vi "Check LM Buffer.vi"(8 "error in (no error)":errorcluster, 10 "SLAM In":T1, 11 "Observed LM Array":T3(array[cluster])) -> (0 "error out":errorcluster, 2 "SLAM Out":T1)   [LabVIEW 2009]
uses:
  Controls/SLAM.ctl
  <vilib>/Analysis/Matrix/Datatypes/RealMatrix.ctl
  cRIO/Functional Global Variables/Actions for FG's.ctl
  <vilib>/Analysis/Matrix/NI_Matrix.lvlib
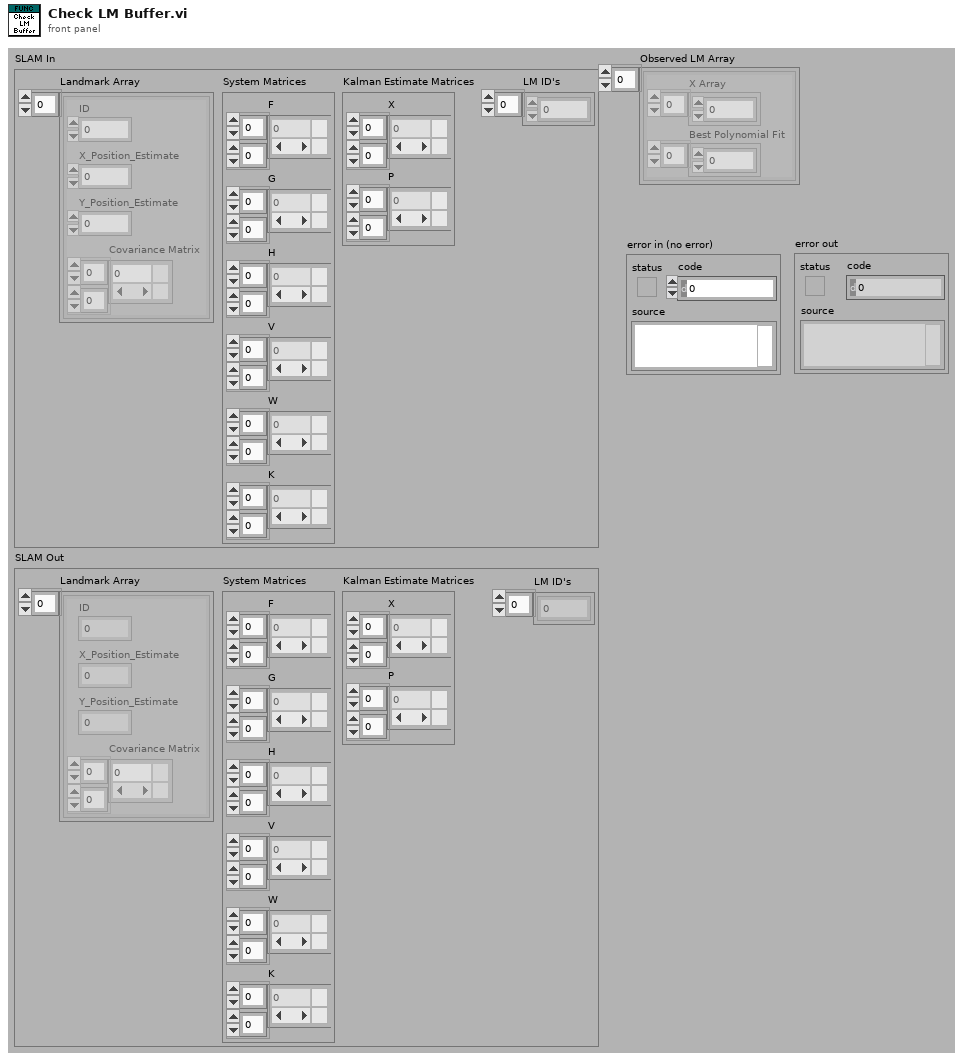
[diagram p1: front panel]
types:
  T1 = typedef "SLAM.ctl" = cluster{"Landmark Array":cluster{"ID":dbl, "X_Position_Estimate":dbl, "Y_Position_Estimate":dbl, "Covariance Matrix":T2}[], "System Matrices":cluster{"F":T2, "G":T2, "H":T2, "V":T2, "W":T2, "K":T2}, "Kalman Estimate Matrices":cluster{"X":T2, "P":T2}, "LM ID's":dbl[]}
  T2 = typedef "NI_Matrix.lvlib/RealMatrix.ctl" = dbl[][]
  T3 = cluster{"X Array":dbl[], "Best Polynomial Fit":dbl[]}[]
  T4 = typedef "Actions for FG's.ctl" = enum16{"Read", "Write"}
  T5 = cluster{"ID":dbl, "X_Position_Estimate":dbl, "Y_Position_Estimate":dbl, "Covariance Matrix":T2}[]
  T6 = cluster{"ID":dbl, "X_Position_Estimate":dbl, "Y_Position_Estimate":dbl, "Covariance Matrix":T2}
  T7 = cluster{"X Array":dbl[], "Best Polynomial Fit":dbl[], "Times Observed":dbl, "Times Not Observed":dbl}[]
  T8 = cluster{"X Array":dbl[], "Best Polynomial Fit":dbl[], "Times Observed":dbl, "Times Not Observed":dbl}
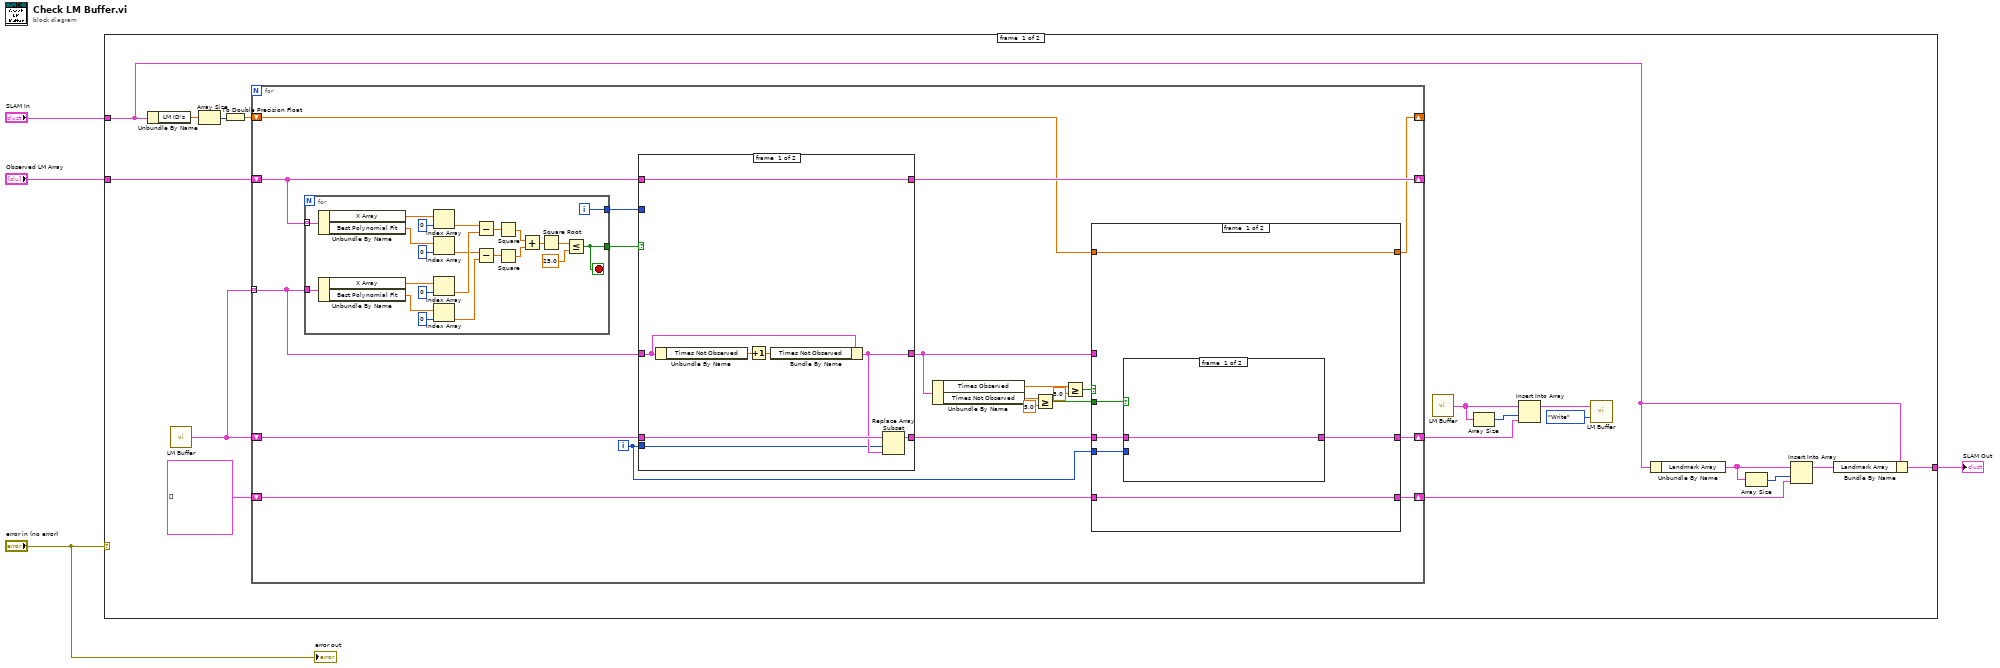
[diagram p0: block diagram]
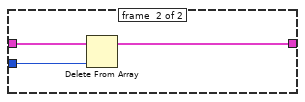
[diagram p2: hidden frame]
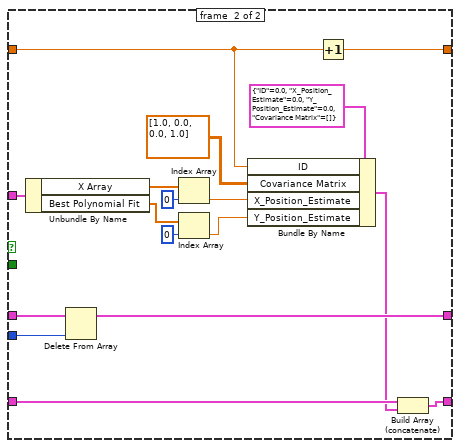
[diagram p3: hidden frame]
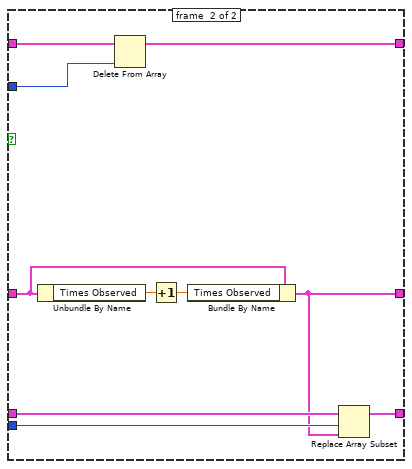
[diagram p4: hidden frame]
diagram:
  n1 = case shown="No Error" "error in (no error)" {
    tunnel: "Observed LM Array" -> [w19 _]
    tunnel: "SLAM In" -> [w7 _]
    tunnel: [w5 _] -> w2
    frame #0 {
      n2 = Unbundle By Name(w7) -> ("LM ID's"=w18:dbl[])
      n3 = call "LM Buffer.vi"() -> ("LM Buffer Out"=w21:T7)  [unwired: 2 in]
      n4 = Array Size(array=w18) -> (size(s)=w17:i32)
      n5 = To Double Precision Float(number=w17) -> (double precision float=w16:dbl)
      n6 = for {
        shift-right: [w38] -> _
        shift-left: w19 -> [w40]
        shift-right: [w30] -> w13
        shift-left: w21 -> [w27]
        shift-right: [w22] -> w8
        shift-left: T5 [] ("Landmark Array") -> [w29]
        tunnel: w21 -> [w28] mode=indexing
        shift-right: [w23] -> _
        shift-left: w16 -> [w24]
        i -> [w25]
        n7 = for {
          tunnel: w28 -> [w109]
          tunnel: w40 -> [w93] mode=indexing
          tunnel: [w95] -> w41
          tunnel: [w94] -> w39
          i -> [w94]
          stop <- w95 stop-if-true
          n8 = Unbundle By Name(w93) -> ("X Array"=w90:dbl[], "Best Polynomial Fit"=w89:dbl[])
          n9 = Unbundle By Name(w109) -> ("X Array"=w106:dbl[], "Best Polynomial Fit"=w105:dbl[])
          n10 = Index Array(array=w90, index=0) -> (element=w88:dbl)
          n11 = Index Array(array=w89, index=0) -> (element=w87:dbl)
          n12 = Index Array(array=w106, index=0) -> (element=w97:dbl)
          n13 = Index Array(array=w105, index=0) -> (element=w96:dbl)
          n14 = Subtract(x=w88, y=w97) -> (x-y=w99:dbl)
          n15 = Subtract(x=w87, y=w96) -> (x-y=w98:dbl)
          n16 = Square(x=w99) -> (x^2=w100:dbl)
          n17 = Square(x=w98) -> (x^2=w101:dbl)
          n18 = Add(x=w100, y=w101) -> (x+y=w102:dbl)
          n19 = Square Root(x=w102) -> (sqrt(x)=w103:dbl)
          n20 = Less Or Equal?(x=w103, y=25.0) -> (x <= y?=w95:bool)
        }
        n21 = case shown="True" w41 {
          tunnel: w28 -> [w73 w86]
          tunnel: [w70 w77] -> w32
          tunnel: w40 -> [w76 w83]
          tunnel: w39 -> [_ w82]
          tunnel: [w76 w81] -> w38
          tunnel: w27 -> [w72 w80]
          tunnel: w25 -> [w69 w79]
          tunnel: [w71 w78] -> w26
          frame #0 {
            n22 = Unbundle By Name(w73) -> ("Times Not Observed"=w74:dbl)
            n23 = Increment(x=w74) -> (x+1=w75:dbl)
            n24 = Bundle By Name(cluster=w73, "Times Not Observed"=w75) -> (w70:T8)
            n25 = Replace Array Subset(array=w72, new element=w70, index=w69) -> (w71:T7)
          }
          frame #1 {
            n26 = Unbundle By Name(w86) -> ("Times Observed"=w84:dbl)
            n27 = Delete From Array(array=w83, index=w82) -> (array with subset deleted=w81:T3)  [unwired: 1 in, 1 out]
            n28 = Increment(x=w84) -> (x+1=w85:dbl)
            n29 = Bundle By Name(cluster=w86, "Times Observed"=w85) -> (w77:T8)
            n30 = Replace Array Subset(array=w80, new element=w77, index=w79) -> (w78:T7)
          }
        }
        n31 = Unbundle By Name(w32) -> ("Times Observed"=w37:dbl, "Times Not Observed"=w34:dbl)
        n32 = Greater Or Equal?(x=w34, y=5.0) -> (x >= y?=w31:bool)
        n33 = Greater Or Equal?(x=w37, y=5.0) -> (x >= y?=w33:bool)
        n34 = case shown="True" w33 {
          tunnel: w32 -> [_ w68]
          tunnel: w31 -> [w47 _]
          tunnel: w26 -> [w45 w67]
          tunnel: w25 -> [w46 w66]
          tunnel: [w44 w65] -> w30
          tunnel: w29 -> [w42 w64]
          tunnel: w24 -> [w43 w55]
          tunnel: [w43 w54] -> w23
          tunnel: [w42 w52] -> w22
          frame #0 {
            n35 = case shown="True" w47 {
              tunnel: w46 -> [_ w51]
              tunnel: w45 -> [w48 w50]
              tunnel: [w48 w49] -> w44
              frame #0 {
              }
              frame #1 {
                n36 = Delete From Array(array=w50, index=w51) -> (array with subset deleted=w49:T7)  [unwired: 1 in, 1 out]
              }
            }
          }
          frame #1 {
            n37 = Unbundle By Name(w68) -> ("X Array"=w61:dbl[], "Best Polynomial Fit"=w60:dbl[])
            n38 = Delete From Array(array=w67, index=w66) -> (array with subset deleted=w65:T7)  [unwired: 1 in, 1 out]
            n39 = Index Array(array=w61, index=0) -> (element=w56:dbl)
            n40 = Index Array(array=w60, index=0) -> (element=w57:dbl)
            n41 = Bundle By Name(cluster=T6 {"ID"=0.0, "X_Position_Estimate"=0.0, "Y_Position_Estimate"=0.0, "Covariance Matrix"=[]} ("Landmarks"), "ID"=w55, "Covariance Matrix"=T2 [[1.0, 0.0], [0.0, 1.0]], "X_Position_Estimate"=w56, "Y_Position_Estimate"=w57) -> (w53:T6)
            n42 = Increment(x=w55) -> (x+1=w54:dbl)
            n43 = Build Array (concatenate)(w64, w53) -> (w52:T5)
          }
        }
      }
      n44 = call "LM Buffer.vi"() -> ("LM Buffer Out"=w15:T7)  [unwired: 2 in]
      n45 = Array Size(array=w15) -> (size(s)=w14:i32)
      n46 = Insert Into Array(array=w15, index=w14, new element=w13) -> (w11:T7)
      n47 = call "LM Buffer.vi"("FG Action (Read)"=Actions_for_FG's."Write", "LM Buffer In"=w11) -> ()  [unwired: 1 out]
      n48 = Unbundle By Name(w7) -> ("Landmark Array"=w9:T5)
      n49 = Array Size(array=w9) -> (size(s)=w10:i32)
      n50 = Insert Into Array(array=w9, index=w10, new element=w8) -> (w6:T5)
      n51 = Bundle By Name(cluster=w7, "Landmark Array"=w6) -> (w5:T1)
    }
    frame #1 {
    }
  }
  "SLAM Out" <- w2
  "error out" <- "error in (no error)"
